vi "Open CSM FP.vi"(7 "Current Module(\"\" to generate a ID)":string, 8 "error in (no error)":errorcluster, 11 "CSM":string) -> (0 "error out":errorcluster)   [LabVIEW 2017, in "csm-tool-support.lvlib"]
doc: "-- <b>输入控件</b> --\n- <b>Current Module(\"\" to generate a ID)</b>:\nThe Argument string to add to the state. The default is an empty string. If Argument is an empty string then State will be returned to the output.\n- <b>error in (no error)</b>:\n- <B>error in</B> can accept error information wired from VIs previously called. Use this information to decide if any functionality should be bypassed in the event of errors from other VIs.\n\nRight-click the <B>error in</B> control on the front panel and select <B>Explain Error</B> or <B>Explain Warning</B> from the shortcut menu for more information about the error.\n- <b>CSM</b>:\n\n\n-- <b>输出控件</b> --\n- <b>error out</b>:\n- <B>error in</B> can accept error information wired from VIs previously called. Use this information to decide if any functionality should be bypassed in the event of errors from other VIs.\n\nRight-click the <B>error in</B> control on the front panel and select <B>Explain Error</B> or <B>Explain Warning</B> from the shortcut menu for more information about the error."
uses:
  csm-tool-support.lvlib
  Communicable State Machine.lvlib
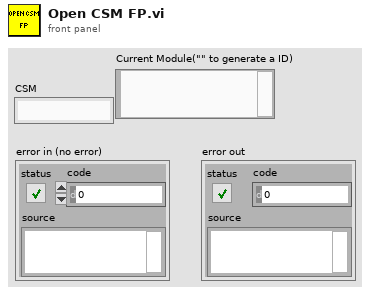
[diagram p1: front panel]
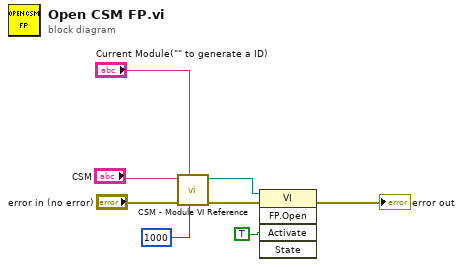
[diagram p0: block diagram]
diagram:
  n1 = call "CSM - Module VI Reference.vi"("Response Timeout(5000ms)"=1000, "Current Module(\"\" to generate a ID)"="Current Module(\"\" to generate a ID)", "error in (no error)"="error in (no error)", "CSM"="CSM") -> ("error out"=w5:errorcluster, "CSM Module VIRef"=w4:refnum<vi>)  [unwired: 6 in]
  n2 = invoke on="Invoke Node" class="VI" method="FP.Open"(reference=w4, error in=w5, "Activate"=TRUE ("Activate?")) -> (error out=→"error out":errorcluster)  [unwired: 2 in, 4 out]
